vi "BREMBO_ANDON_ SHIFTWISE_DATE.vi"(10 "shift":i32, 11 "sHIFT":string) -> (3 "date/time string":string)   [LabVIEW 2017]
uses:
  <vilib>/addons/database/Auxilliary.llb/DB Tools Format Datetime String (Time Stamp).vi
  <vilib>/addons/database/NI_Database_API.lvlib
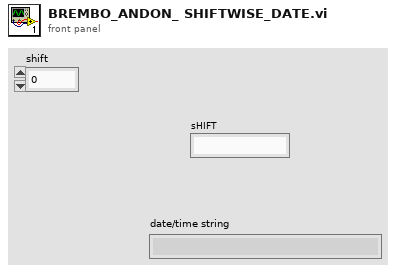
[diagram p1: front panel]
types:
  T1 = typedef "LVDateTimeRec.ctl" = cluster{"fractional second":dbl, "second":i32, "minute":i32, "hour":i32, "day of month":i32, "month":i32, "year":i32, "day of week":i32, "day of year":i32, "DST":i32}
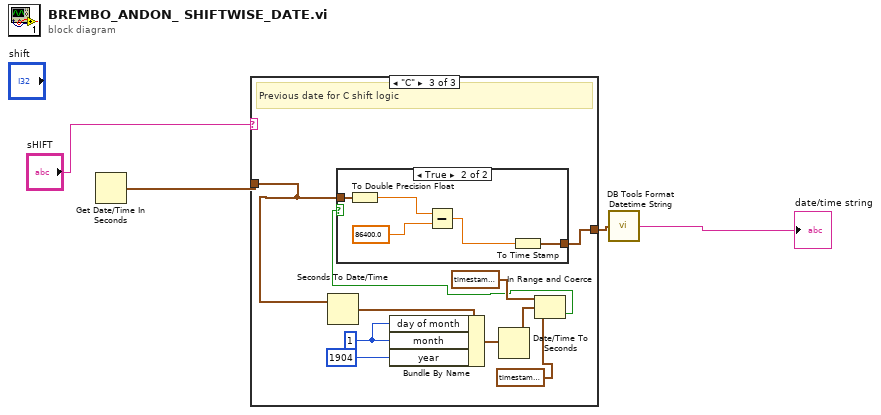
[diagram p0: block diagram]
diagram:
  n1 = Get Date/Time In Seconds() -> (seconds since 1Jan1904=w3:timestamp)
  n2 = case shown="\"C\"" "sHIFT" {
    tunnel: w3 -> [w5 w6 w11]
    tunnel: [w5 w6 w16] -> w2
    frame "A", Default {
    }
    frame "B" {
    }
    frame "C" {
      w12 = 1 ("day of month")
      # "Previous date for C shift logic"
      n3 = Seconds To Date/Time(time stamp (now)=w11) -> (date time rec=w13:T1)  [unwired: 1 in]
      n4 = Bundle By Name(cluster=w13, "day of month"=w12, "month"=w12, "year"=1904) -> (w15:T1)
      n5 = Date/Time To Seconds(2:w15) -> (0:w10:timestamp)  [unwired: 1 in]
      n6 = In Range and Coerce(upper limit=timestamp(12600 s since 1904-01-01), x=w10, lower limit=timestamp(-19800 s since 1904-01-01)) -> (In Range?=w7:bool)  [unwired: 1 out]
      n7 = case shown="True" w7 {
        tunnel: [w17 w19] -> w16
        tunnel: w11 -> [w17 w18]
        frame False {
        }
        frame True {
          n8 = To Double Precision Float(number=w18) -> (double precision float=w22:dbl)
          n9 = Subtract(x=w22, y=86400.0) -> (x-y=w20:dbl)
          n10 = To Time Stamp(1:w20) -> (0:w19:timestamp)
        }
      }
    }
  }
  n11 = call-poly <vilib>:"DB Tools Format Datetime String.vi"("time stamp"=w2) -> ("date/time string"=→"date/time string":string)
